vi "Software Update HCC Get Latest Folder Path.vi"(7 "Machine Type":enum16{"2015", "Viper/Hawk"}(ring), 8 "Error In":errorcluster, 10 "Standard Newfi Location":path=path "\\\\3.67.38.12\\share/AP1_Library/Executables/Washer Hcc/HCC Files/2015 Laundry", 11 "Standard 2015 Location":path=path "\\\\3.67.38.12\\share/AP1_Library/Executables/Washer Hcc/HCC Files/2015 Laundry") -> (0 "Error Out":errorcluster, 3 "Latest Path":path)   [LabVIEW 2014]
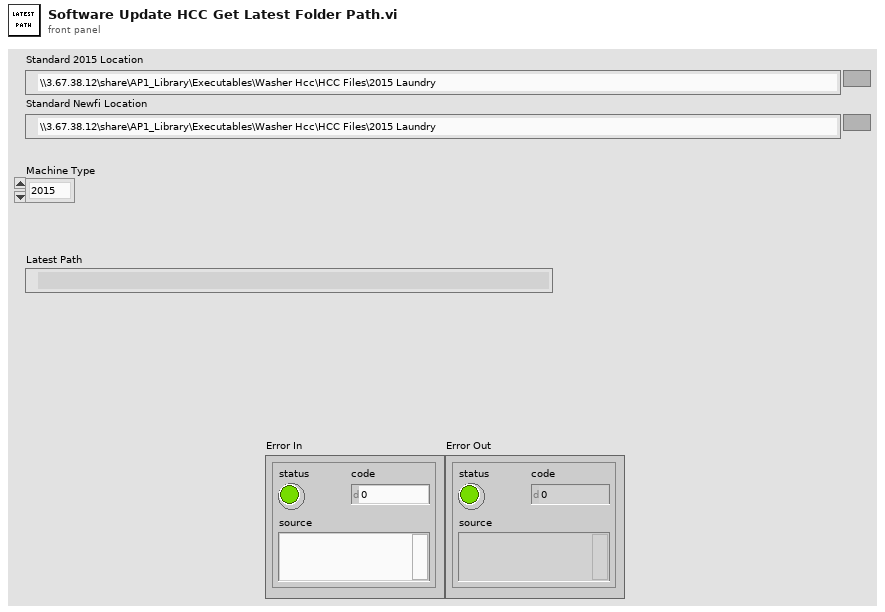
[diagram p1: front panel]
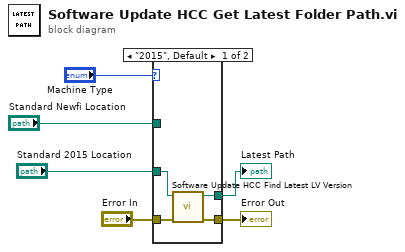
[diagram p0: block diagram]
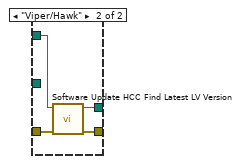
[diagram p2: hidden frame]
diagram:
  n1 = case shown="\"2015\", Default" "Machine Type" {
    tunnel: "Error In" -> [w10 w14]
    tunnel: [w9 w13] -> w5
    tunnel: "Standard Newfi Location" -> [_ w12]
    tunnel: [w7 w11] -> w2
    tunnel: "Standard 2015 Location" -> [w8 _]
    frame "2015", Default {
      n2 = call "Software Update HCC Find Latest LV Version.vi"("Error In"=w10, "Standard Newfi Location"=w8) -> ("Error Out"=w9:errorcluster, "appended path"=w7:path)  [unwired: 8 in]
    }
    frame "Viper/Hawk" {
      n3 = call "Software Update HCC Find Latest LV Version.vi"("Error In"=w14, "Standard Newfi Location"=w12) -> ("Error Out"=w13:errorcluster, "appended path"=w11:path)  [unwired: 8 in]
    }
  }
  "Latest Path" <- w2
  "Error Out" <- w5
